vi "Read Elements of HTML&PDFnames.vi"(8 "error in (no error)":errorcluster, 11 "Folder_Mgmt":refnum<class "Folder_Mgmt.lvclass">) -> (0 "error out":errorcluster, 2 "PDFnames":string[](array[string]), 3 "Folder_Mgmt 2":refnum<class "Folder_Mgmt.lvclass">)   [LabVIEW 2016, in "Folder_Mgmt.lvclass"]
uses:
  Folder_Mgmt.lvclass
  Folder_Mgmt.lvclass/Folder_Mgmt.ctl
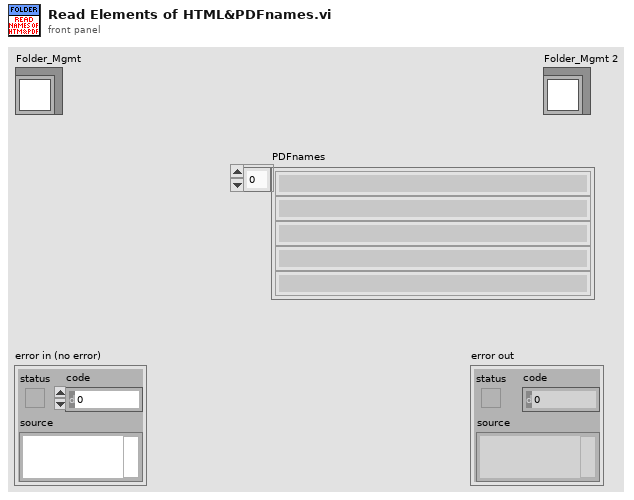
[diagram p1: front panel]
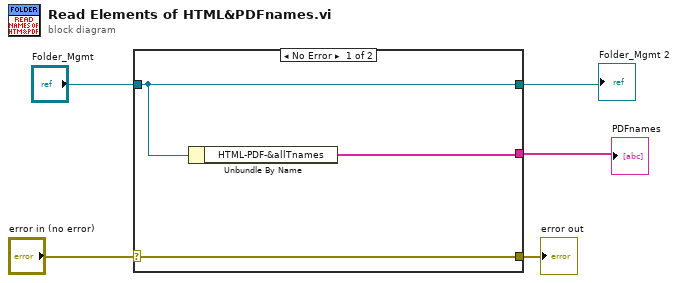
[diagram p0: block diagram]
diagram:
  n1 = case shown="No Error" "error in (no error)" {
    selector: "error in (no error)" -> [w8 w9]
    tunnel: [w8 w9] -> w4
    tunnel: [w7 w10] -> w1
    tunnel: "Folder_Mgmt" -> [w7 w10]
    tunnel: [w6 _] -> w3
    frame No Error {
      n2 = Unbundle By Name(w7) -> ("HTML-PDF-&allTnames"=w6:string[])
    }
    frame Error {
    }
  }
  "error out" <- w4
  "PDFnames" <- w3
  "Folder_Mgmt 2" <- w1
